vi "xijk_image_overlay message.vi"(6 "Group":string="message", 8 "error in":errorcluster, 10 "message number":i32, 11 "Image In":T1) -> (0 "error out":errorcluster, 3 "Image Out (duplicate)":T1)   [LabVIEW 2010]
uses:
  <vilib>/vision/Image Controls.llb/IMAQ Image.ctl
panel:
  in  "Font, Size & Style":T2={"Desired Font (Application)"=enum."Application Font", "[User-specified Font]"={"Font Name"="", "Size"=14, "Strikeout?"=FALSE, "Italic?"=FALSE, "Underline?"=FALSE, "Outline?"=FALSE, "Shadow?"=FALSE, "Bold?"=TRUE, "Rotation Angle"=0.0}, "Horizontal Alignment"=0, "Vertical Alignment"=0} {"Horizontal Alignment" items=["Left", "Center", "Right"]; "Vertical Alignment" items=["Bottom", "Top", "Baseline"]}
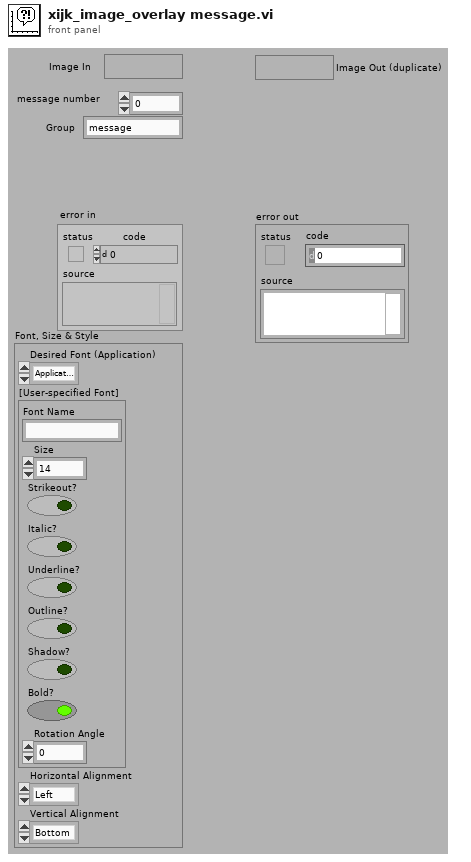
[diagram p1: front panel]
types:
  T1 = typedef "IMAQ Image.ctl" = refnum<image>
  T2 = cluster{"Desired Font (Application)":enum16{"User-specified Font", "Application Font", "System Font", "Dialog Font"}, "[User-specified Font]":cluster{"Font Name":string, "Size":i16, "Strikeout?":bool, "Italic?":bool, "Underline?":bool, "Outline?":bool, "Shadow?":bool, "Bold?":bool, "Rotation Angle":dbl}, "Horizontal Alignment":i16, "Vertical Alignment":i16}
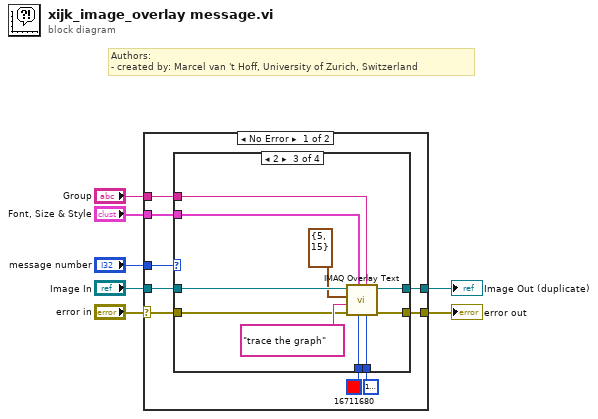
[diagram p0: block diagram]
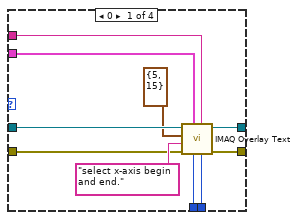
[diagram p2: hidden frame]
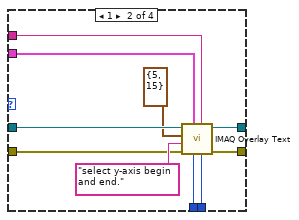
[diagram p3: hidden frame]
diagram:
  # "Authors: \n- created by: Marcel van 't Hoff, University of Zurich, Switzerland"
  n1 = case shown="No Error" "error in" {
    selector: "error in" -> [w11 w48]
    tunnel: "Font, Size & Style" -> [w16 _]
    tunnel: [w15 w48] -> w6
    tunnel: [w14 w49] -> w5
    tunnel: "Image In" -> [w13 w49]
    tunnel: "message number" -> [w12 _]
    tunnel: "Group" -> [w8 _]
    frame No Error {
      n2 = case shown="2" w12 {
        tunnel: w13 -> [w26 w36 w46 w47]
        tunnel: [w25 w35 w45 w47] -> w14
        tunnel: w16 -> [w21 w31 w41 _]
        tunnel: [w22 w32 w42 _] -> w15
        tunnel: w11 -> [w20 w30 w40 _]
        tunnel: u32 16711680 ("Text Color (black)") -> [w19 w29 w39 _]
        tunnel: u32 16777226 ("BG Color (Transparent)") -> [w18 w28 w38 _]
        tunnel: w8 -> [w17 w27 w37 _]
        frame 0 {
          n3 = call "IMAQ Overlay Text"("BG Color (Transparent)"=w18, "Group"=w17, "Text Color (black)"=w19, "Font, Size & Style"=w21, "error in (no error)"=w20, "String"="select x-axis begin and end.", "Origin"=cluster{"X":i32, "Y":i32} {"X"=5, "Y"=15}, "Image"=w26) -> ("error out"=w22:errorcluster, "Image Out"=w25:T1)  [unwired: 2 in]
        }
        frame 1 {
          n4 = call "IMAQ Overlay Text"("BG Color (Transparent)"=w28, "Group"=w27, "Text Color (black)"=w29, "Font, Size & Style"=w31, "error in (no error)"=w30, "String"="select y-axis begin and end.", "Origin"=cluster{"X":i32, "Y":i32} {"X"=5, "Y"=15}, "Image"=w36) -> ("error out"=w32:errorcluster, "Image Out"=w35:T1)  [unwired: 2 in]
        }
        frame 2 {
          n5 = call "IMAQ Overlay Text"("BG Color (Transparent)"=w38, "Group"=w37, "Text Color (black)"=w39, "Font, Size & Style"=w41, "error in (no error)"=w40, "String"="trace the graph", "Origin"=cluster{"X":i32, "Y":i32} {"X"=5, "Y"=15}, "Image"=w46) -> ("error out"=w42:errorcluster, "Image Out"=w45:T1)  [unwired: 2 in]
        }
        frame Default {
        }
      }
    }
    frame Error {
    }
  }
  "error out" <- w6
  "Image Out (duplicate)" <- w5
